vi "FahrzustandSchaltung.vi"(4 "Sensoren":dbl[](array[numeric]), 5 "Geschwindigkeitsmultiplikator":dbl) -> (0 "PWM Motor":dbl, 1 "PWM Lenkung":dbl, 2 "Linefollow_Array":bool[](array[boolean]))   [LabVIEW 2016]
uses:
  Control/FolgenEnum.ctl
  <vilib>/myRIO/Instrument Drivers/Onboard IO/DIO/typedefs/DIO Reference.ctl
  <vilib>/myRIO/Common/Instrument Driver Framework/Utilities/typedefs/myRIO Generic Hardware Reference.ctl
  <vilib>/myRIO/Common/Instrument Driver Framework/Utilities/typedefs/Hardware Version Enum.ctl
  <vilib>/myRIO/Common/Instrument Driver Framework/Utilities/typedefs/myRIO v1.0 Reference.ctl
  <vilib>/myRIO/Common/Instrument Driver Framework/Utilities/typedefs/Generic FPGA Reference.ctl
  <vilib>/myRIO/Common/Instrument Driver Framework/myRIO v1.0/DIO/typedefs/DIO Channels List.ctl
  <vilib>/myRIO/Common/Instrument Driver Framework/myRIO v1.0/DIO/typedefs/DIO Channels Enum.ctl
  <vilib>/userdefined/High Color/nirio_resource_hc.ctl
  <vilib>/myRIO/Common/Instrument Driver Framework/Utilities/vis/Is FPGA Ref Available.vi
  <vilib>/myRIO/Common/Instrument Driver Framework/myRIO v1.0/DIO/vis/myRIO v1.1 Open DIO.vi
  <vilib>/myRIO/Instrument Drivers/Onboard IO/DIO/vis/Write.vi
  <vilib>/myRIO/Common/Instrument Driver Framework/Utilities/vis/Validate Channels.vi
  <vilib>/myRIO/Common/Instrument Driver Framework/myRIO v1.0/DIO/vis/myRIO v1.0 Reserve DIO.vi
  <vilib>/myRIO/Common/Instrument Driver Framework/myRIO v1.0/Resource Manager/vis/myRIO v1.0 Reserve Channel List.vi
  <vilib>/myRIO/Common/Instrument Driver Framework/myRIO v1.0/DIO/vis/myRIO v1.0 Build MUX Configuration DIO.vi
  <vilib>/myRIO/Common/Instrument Driver Framework/myRIO v1.0/Resource Manager/vis/myRIO v1.0 Reserve Channel.vi
  <vilib>/myRIO/Common/Instrument Driver Framework/myRIO v1.0/Resource Manager/vis/myRIO v1.0 Unreserve Channel.vi
  <vilib>/myRIO/Common/Instrument Driver Framework/myRIO v1.0/Resource Manager/vis/myRIO v1.0 Create Configuration List.vi
  <vilib>/myRIO/Common/Instrument Driver Framework/myRIO v1.0/Resource Manager/vis/myRIO v1.0 Build Mutex Name.vi
  <vilib>/Utility/VariantDataType/GetNumericInfo.vi
  <vilib>/Utility/error.llb/Error Cluster From Error Code.vi
  <vilib>/myRIO/Common/Instrument Driver Framework/myRIO v1.0/myRIO v1.1 Open.vi
  <vilib>/myRIO/Common/Instrument Driver Framework/Utilities/vis/IO Manager.vi
  <vilib>/myRIO/Common/Instrument Driver Framework/Utilities/vis/Configuration Manager.vi
  <vilib>/myRIO/Common/Instrument Driver Framework/myRIO v1.0/Resource Manager/vis/myRIO v1.0 Configure IO.vi
  <vilib>/myRIO/Common/Instrument Driver Framework/myRIO v1.0/myRIO v1.0 Close.vi
  <vilib>/myRIO/Common/Instrument Driver Framework/myRIO v1.0/DIO/vis/myRIO v1.0 Write DIO.vi
  <vilib>/myRIO/Express VI/Onboard IO/DO/DO Express VI.xnode
  <vilib>/myRIO/Instrument Drivers/Onboard IO/DIO/vis/myRIO DIO Open.xnode
  <vilib>/myRIO/Instrument Drivers/Onboard IO/DIO/DIO.lvlib
panel:
  out "TimeStartüberholen":u32
  out "TimeStartFollow":u32
  out "Position Strecke":dbl
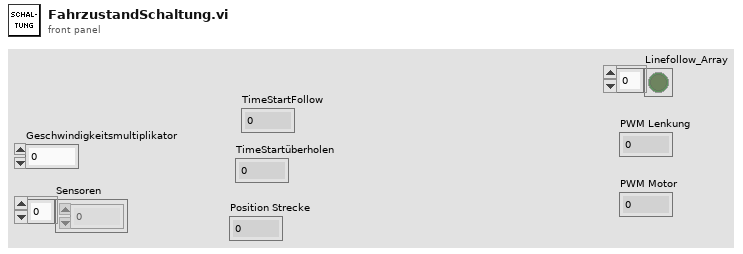
[diagram p1: front panel]
types:
  T1 = typedef "FolgenEnum.ctl" = enum16{"Suchen", "Folgen", "überholen"}
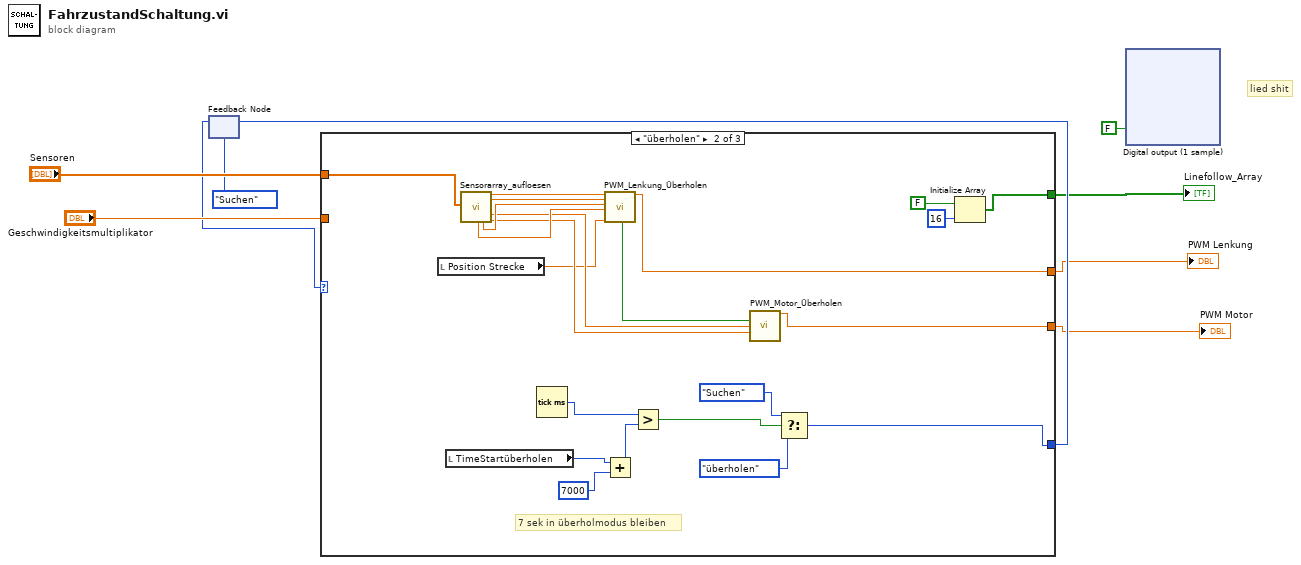
[diagram p0: block diagram]
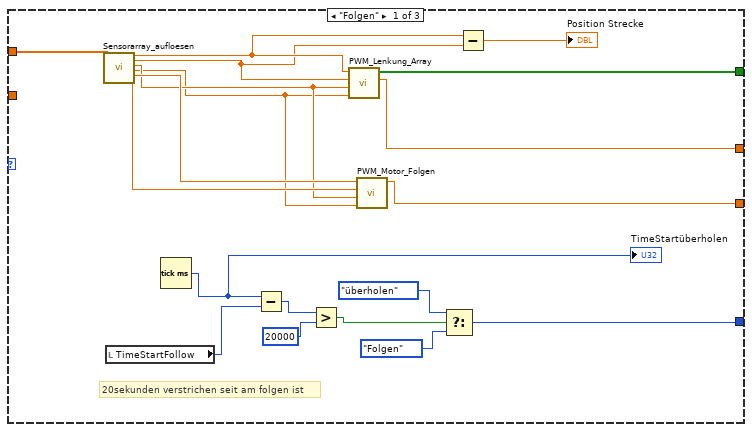
[diagram p2: hidden frame]
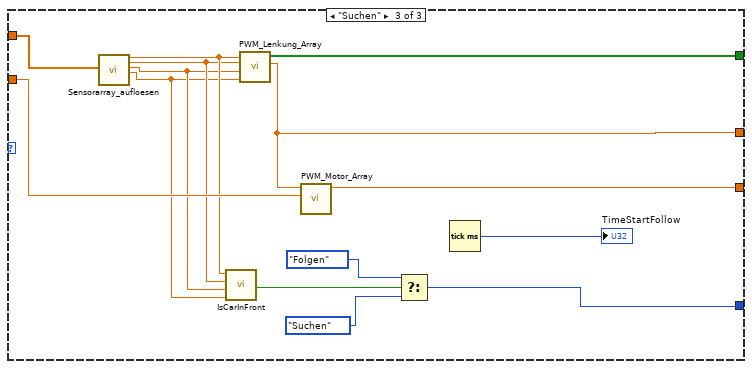
[diagram p3: hidden frame]
diagram:
  # "lied shit"
  n1 = feedback #1(FolgenEnum."Suchen") -> (w5:T1)
  n2 = case shown="\"überholen\"" w5 {
    tunnel: "Geschwindigkeitsmultiplikator" -> [_ _ w63]
    tunnel: "Sensoren" -> [w28 w42 w64]
    tunnel: [w23 w41 w62] -> w3
    tunnel: [w21 w30 w61] -> w2
    tunnel: [w22 w40 w60] -> w4
    tunnel: [w11 w32 w52] -> w7
    frame "Folgen" {
      # "20sekunden verstrichen seit am folgen ist"
      n3 = call "Sensorarray_aufloesen.vi"("Array"=w28) -> (14:w20:dbl, "vorne links"=w19:dbl, "schräg rechts"=w25:dbl, "schräg links"=w24:dbl, "gerade rechts"=w27:dbl, "gerade links"=w26:dbl)  [unwired: 11 in, 2 out]
      n4 = local read "TimeStartFollow"() -> (w17:u32)
      n5 = Tick Count (ms)() -> (millisecond timer value=w10:u32)
      "TimeStartüberholen" <- w10
      n6 = Subtract(x=w10, y=w17) -> (x-y=w16:u32)
      n7 = Greater?(x=w16, y=u32 20000) -> (0:w14:bool)
      n8 = call "PWM_Lenkung_Array.vi"("schräg links"=w24, "schräg rechts"=w25, "vorne links"=w19, "vorne rechts"=w20) -> ("PWM Lenkung"=w22:dbl, "Linefollow_Array"=w21:bool[])  [unwired: 4 in, 1 out]
      n9 = call "PWM_Motor_Folgen.vi"("Sensor gerade rechts"=w27, "Sensor gerade links"=w26, "Sensor schräg rechts"=w25, "Sensor schräg links"=w24) -> ("PWM Motor"=w23:dbl)  [unwired: 6 in]
      n10 = Select(t=FolgenEnum."überholen", s=w14, f=FolgenEnum."Folgen") -> (s? t:f=w11:T1)
      n11 = Subtract(x=w20, y=w19) -> (x-y=→"Position Strecke":dbl)
    }
    frame "überholen" {
      # "7 sek in überholmodus bleiben"
      n12 = local read "Position Strecke"() -> (w43:dbl)
      n13 = local read "TimeStartüberholen"() -> (w38:u32)
      n14 = call "Sensorarray_aufloesen.vi"("Array"=w42) -> ("hinten links"=w47:dbl, "hinten rechts"=w48:dbl, 14:w50:dbl, "vorne links"=w49:dbl, "gerade rechts"=w46:dbl, "gerade links"=w45:dbl)  [unwired: 11 in, 2 out]
      n15 = Tick Count (ms)() -> (millisecond timer value=w39:u32)
      n16 = call "PWM_Lenkung_Überholen.vi"("vorne rechts"=w50, "vorne links"=w49, "hinten rechts"=w48, "hinten links"=w47, "Position Strecke"=w43) -> ("Abstand Bande erreicht"=w44:bool, "PWM Lenkung"=w40:dbl)  [unwired: 13 in]
      n17 = Add(x=w38, y=u32 7000) -> (x+y=w37:u32)
      n18 = Greater?(x=w39, y=w37) -> (0:w35:bool)
      n19 = call "PWM_Motor_Überholen.vi"("Abstand Bande erreicht"=w44, "Sensor geradeaus rechts"=w46, "Sensor geradeaus links"=w45) -> ("PWM Motor"=w41:dbl)  [unwired: 12 in]
      n20 = Select(t=FolgenEnum."Suchen", s=w35, f=FolgenEnum."überholen") -> (s? t:f=w32:T1)
      n21 = Initialize Array(FALSE, 16 ("dimension size")) -> (w30:bool[])
    }
    frame "Suchen" {
      n22 = call "Sensorarray_aufloesen.vi"("Array"=w64) -> (14:w59:dbl, "vorne links"=w58:dbl, "schräg rechts"=w57:dbl, "schräg links"=w56:dbl)  [unwired: 11 in, 4 out]
      n23 = call "IsCarInFront.vi"("schräg Links"=w56, "schräg Rechts"=w57, "geradeaus Links"=w58, "geradeaus Rechts"=w59) -> ("IsFollowingAuto"=w55:bool)
      n24 = call "PWM_Lenkung_Array.vi"("schräg links"=w56, "schräg rechts"=w57, "vorne links"=w58, "vorne rechts"=w59) -> ("PWM Lenkung"=w60:dbl, "Linefollow_Array"=w61:bool[])  [unwired: 4 in, 1 out]
      n25 = call "PWM_Motor_Array.vi"("Geschwindigkeit\nmultiplikator"=w63, "PWM Sensor"=w60) -> ("PWM Motor"=w62:dbl)  [unwired: 9 in]
      n26 = Select(t=FolgenEnum."Folgen", s=w55, f=FolgenEnum."Suchen") -> (s? t:f=w52:T1)
      n27 = Tick Count (ms)() -> (millisecond timer value=→"TimeStartFollow":u32)
    }
  }
  "PWM Motor" <- w3
  "PWM Lenkung" <- w4
  "Linefollow_Array" <- w2
  n28 = feedback-in #1(w7) -> ()
  n29 = xnode "Digital output (1 sample)"("A/DIO9 (Pin 29)"=FALSE) -> ()  [unwired: 1 in, 1 out]
